vi "ReadKeithley2614.vi"() -> ()   [LabVIEW 2014]
panel:
  in  "error in (no error)":errorcluster
  out "error out":errorcluster
  out "String 4":string
  in  "String":string
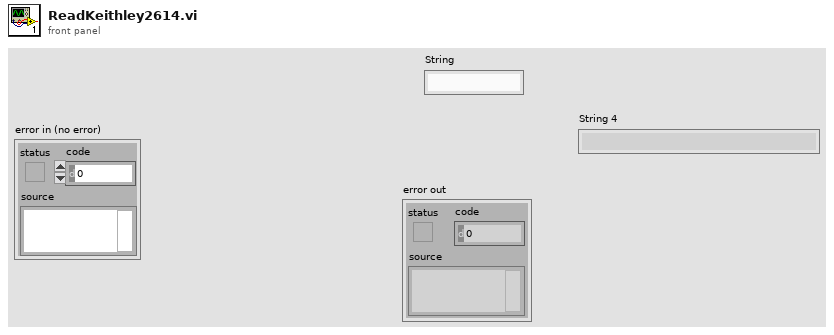
[diagram p1: front panel]
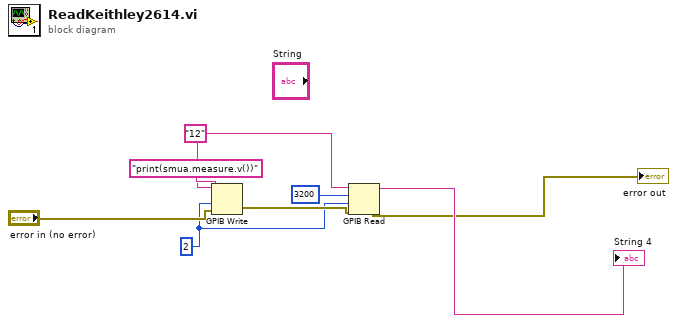
[diagram p0: block diagram]
diagram:
  w1 = 2
  w3 = "12"
  n1 = GPIB Write(0:w3, 1:"print(smua.measure.v())", 2:w1, 3:"error in (no error)") -> (6:w8:errorcluster)  [unwired: 1 in, 1 out]
  n2 = GPIB Read(0:w3, 1:3200, 2:w1, 3:w8) -> (5:→"String 4":string, 7:→"error out":errorcluster)  [unwired: 1 in, 1 out]
